vi "CRYAcquisition Global.vi"() -> ()   [LabVIEW 2013]
panel:
  out "Test Mode":bool
  in  "Old Curve Name":string[](array[string])
  in  "Curve Type":enum16{"Curves", "Values", "Results", "WFM"}(ring)
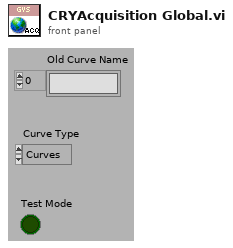
[diagram p1: front panel]
diagram:
